vi "Start Channel Stream.vi"(6 "Channel index":i32, 8 "error in (no error)":errorcluster, 9 "Waveform":waveform(i16), 11 "Pulse Driver in":refnum<class "Pulse Driver.lvclass">) -> (0 "error out":errorcluster, 1 "channel name(s) out":string, 2 "group name out":string, 3 "Pulse Driver out":refnum<class "Pulse Driver.lvclass">)   [LabVIEW 2016, in "Pulse Driver.lvclass"]
uses:
  Pulse Driver.lvclass
  C:/github/NHMFL_Core/Libraries/Instruments/Instrument Driver/Instrument Driver.lvclass
  Pulse Driver.lvclass/Pulse Driver.ctl
  Instrument Driver/Instrument Driver.lvclass/Instrument Driver.ctl
  Read Scaling coefficients.vi
  Read tdms file.vi
  Instrument Driver/Read Channel names.vi
  Instrument Driver/Read Group name.vi
  Write tdms file.vi
  <vilib>/Utility/tdmsutil.llb/TDMS Create Scaling Information (Linear).vi
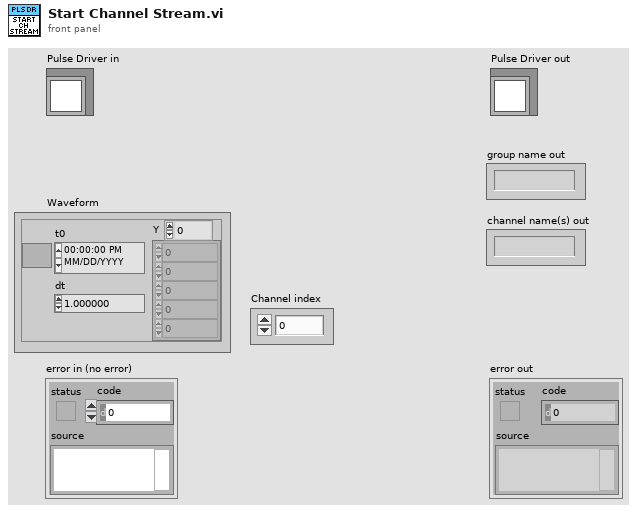
[diagram p1: front panel]
types:
  T1 = cluster{"slope":dbl, "y intercept":dbl, "input source":i32}
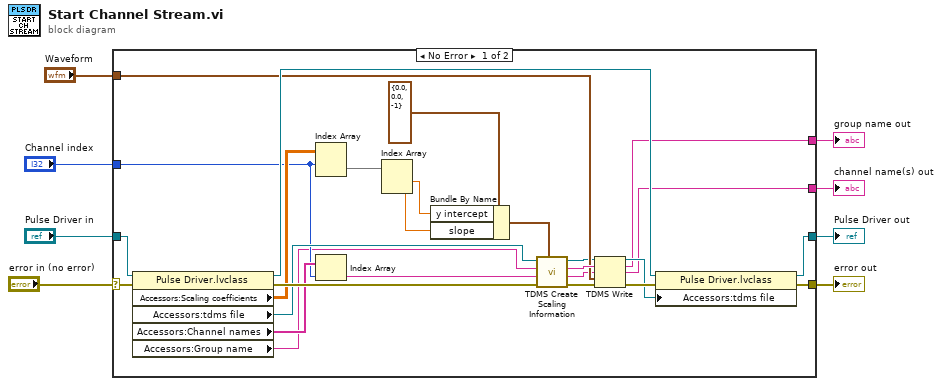
[diagram p0: block diagram]
diagram:
  n1 = case shown="No Error" "error in (no error)" {
    selector: "error in (no error)" -> [w13 w36]
    tunnel: [w14 w36] -> w7
    tunnel: [w17 w35] -> w5
    tunnel: "Pulse Driver in" -> [w34 w35]
    tunnel: "Channel index" -> [w21 _]
    tunnel: "Waveform" -> [w20 _]
    tunnel: [w11 _] -> w2
    tunnel: [w10 _] -> w1
    frame No Error {
      n2 = property class="Pulse Driver.lvclass"(reference=w34, error in=w13) -> (reference out=w33:refnum<class "Pulse Driver.lvclass">, error out=w30:errorcluster, "Accessors:Scaling coefficients"=w27:dbl[][], "Accessors:tdms file"=w28:refnum<k34>, "Accessors:Channel names"=w29:string[], "Accessors:Group name"=w12:string)
      n3 = Index Array(array=w27, index (row)=w21) -> (element=w25:dbl[])  [unwired: 1 in]
      n4 = Index Array(array=w29, index=w21) -> (element=w26:string)
      n5 = Index Array(array=w25) -> (element #1=w32:dbl, element #2=w9:dbl)  [unwired: 2 in]
      n6 = Bundle By Name(cluster=T1 {"slope"=0.0, "y intercept"=0.0, "input source"=-1} ("linear scale"), "y intercept"=w32, "slope"=w9) -> (w31:T1)
      n7 = call-poly <vilib>:"TDMS Create Scaling Information.vi"("linear scale"=w31, "error in (no error)"=w30, "channel name"=w26, "group name"=w12, "tdms file"=w28) -> ("error out"=w23:errorcluster, "channel name out"=w19:string, "group name out"=w22:string, "tdms file out"=w18:refnum<k34>)  [unwired: 2 in, 1 out]
      n8 = TDMS Write(0:w18, 5:w22, 7:w19, 9:w20, 11:w23) -> (4:w15:refnum<k34>, 6:w11:string, 8:w10:string, 15:w16:errorcluster)  [unwired: 1 in]
      n9 = property class="Pulse Driver.lvclass"(reference=w33, error in=w16, "Accessors:tdms file"=w15) -> (reference out=w17:refnum<class "Pulse Driver.lvclass">, error out=w14:errorcluster)
    }
    frame Error {
    }
  }
  "error out" <- w7
  "Pulse Driver out" <- w5
  "channel name(s) out" <- w1
  "group name out" <- w2
